vi "Shift.vi"(8 "error in":errorcluster) -> (0 "error out":errorcluster)   [LabVIEW 2015]
uses:
  Control Button/Save.ctl
  Control Button/Exit.ctl
  <vilib>/addons/database/Connection.llb/DB Tools Open Connec (String).vi
  <vilib>/addons/database/_DB Variant To Data/Database Variant To Data.xnode
  <vilib>/addons/database/NI_Database_API.lvlib
panel:
  in  "To-C 2":timestamp=timestamp(3526421399 s since 1904-01-01) format="%<%H:%M:%S\n%d/%m/%Y>T"
  in  "From-C 2":timestamp=timestamp(3526482600 s since 1904-01-01) format="%<%H:%M:%S\n%d/%m/%Y>T"
  out "error out 2":errorcluster
  out "error out":errorcluster
  out "Shift":string="B"
  in  "To-C 1":timestamp=timestamp(3526421399 s since 1904-01-01) format="%<%H:%M:%S\n%d/%m/%Y>T"
  in  "From-C 1":timestamp=timestamp(3526482600 s since 1904-01-01) format="%<%H:%M:%S\n%d/%m/%Y>T"
  in  "To-B":timestamp=timestamp(3526482599 s since 1904-01-01) format="%<%H:%M:%S\n%d/%m/%Y>T"
  in  "From-B":timestamp=timestamp(3526452000 s since 1904-01-01) format="%<%H:%M:%S\n%d/%m/%Y>T"
  in  "To-A":timestamp=timestamp(3526451999 s since 1904-01-01) format="%<%H:%M:%S\n%d/%m/%Y>T"
  in  "From-A":timestamp=timestamp(3526594200 s since 1904-01-01) format="%<%H:%M:%S\n%d/%m/%Y>T"
  in  "Exit":T1
  in  "Save":T2
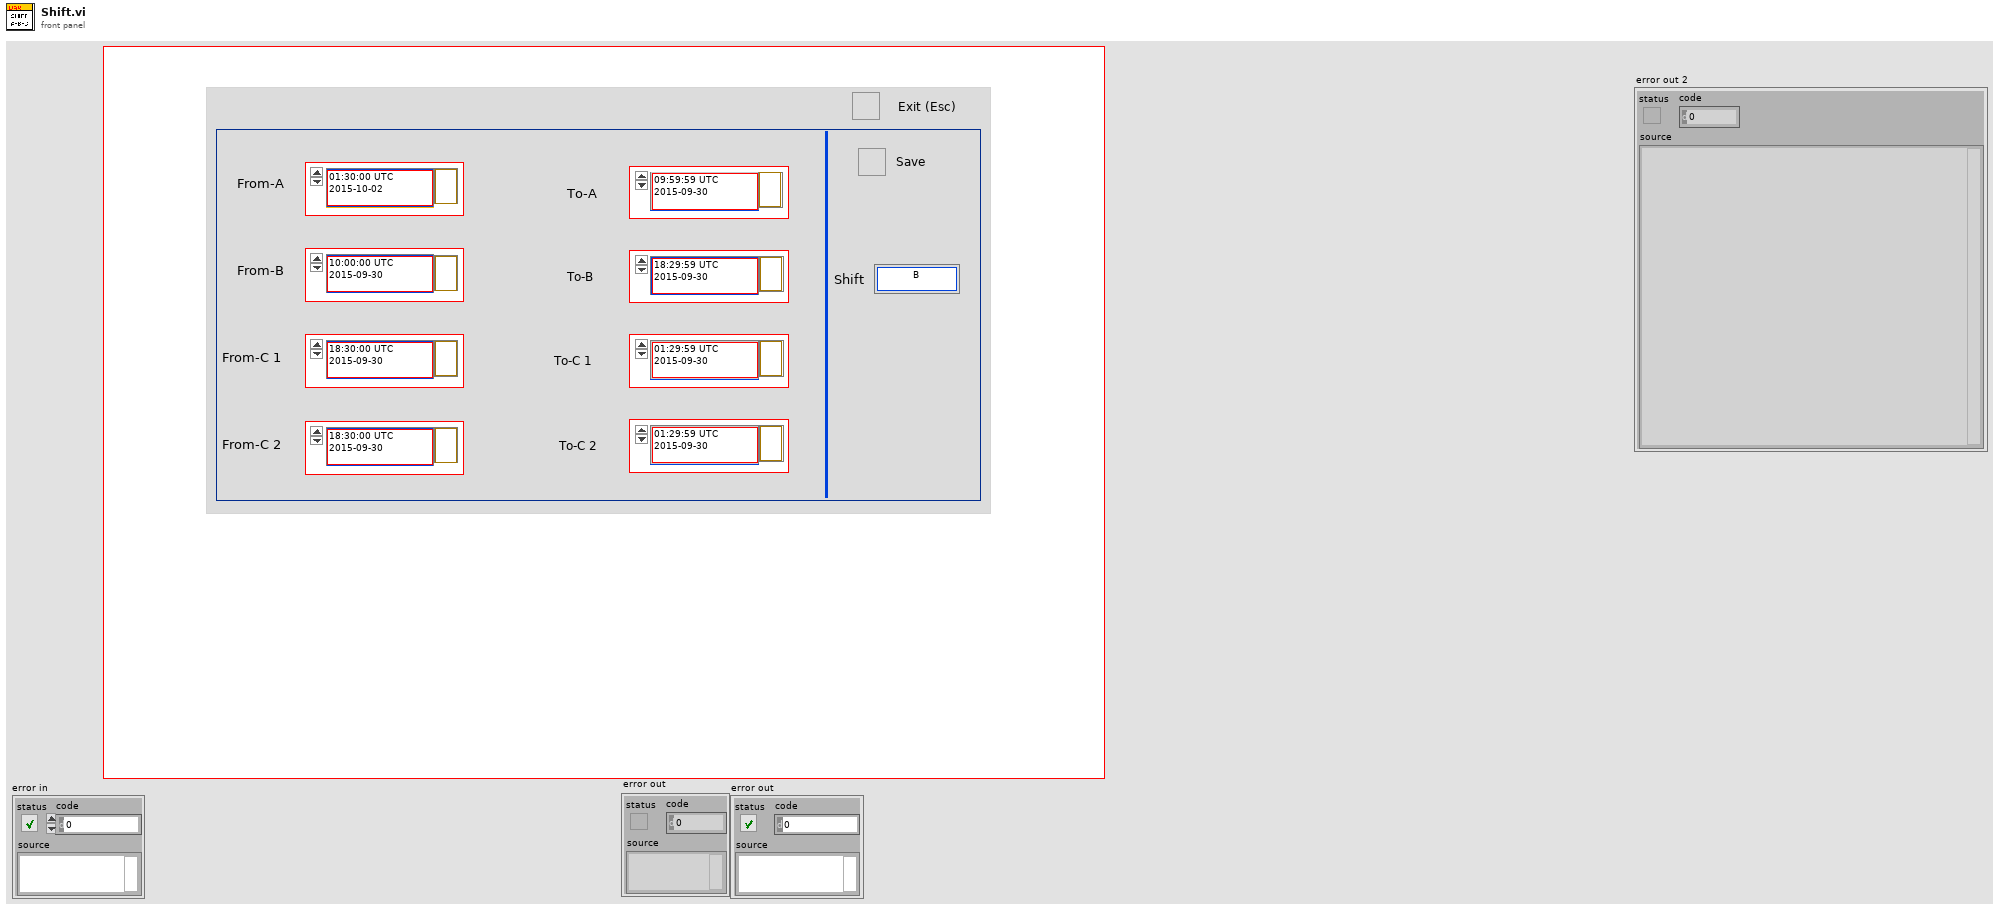
[diagram p1: front panel]
types:
  T1 = typedef "Exit.ctl" = bool
  T2 = typedef "Save.ctl" = bool
  T3 = cluster{"To-A":timestamp, "From-A":timestamp, "From-B":timestamp, "To-B":timestamp, "From-C 1":timestamp, "To-C 1":timestamp, "Shift":string, "To-C 2":timestamp, "From-C 2":timestamp}[]
  T4 = cluster{"To-A":timestamp, "From-A":timestamp, "From-B":timestamp, "To-B":timestamp, "From-C 1":timestamp, "To-C 1":timestamp, "Shift":string, "To-C 2":timestamp, "From-C 2":timestamp}
  T5 = typedef "NI_Database_API.lvlib/Conn ObjectReference.ctl" = refnum<k1>
  T6 = cluster{"To-A":timestamp, "From-A":timestamp, "From-B":timestamp, "To-B":timestamp, "From-C 1":timestamp, "To-C 1":timestamp, "From-C 2":timestamp, "To-C 2":timestamp}
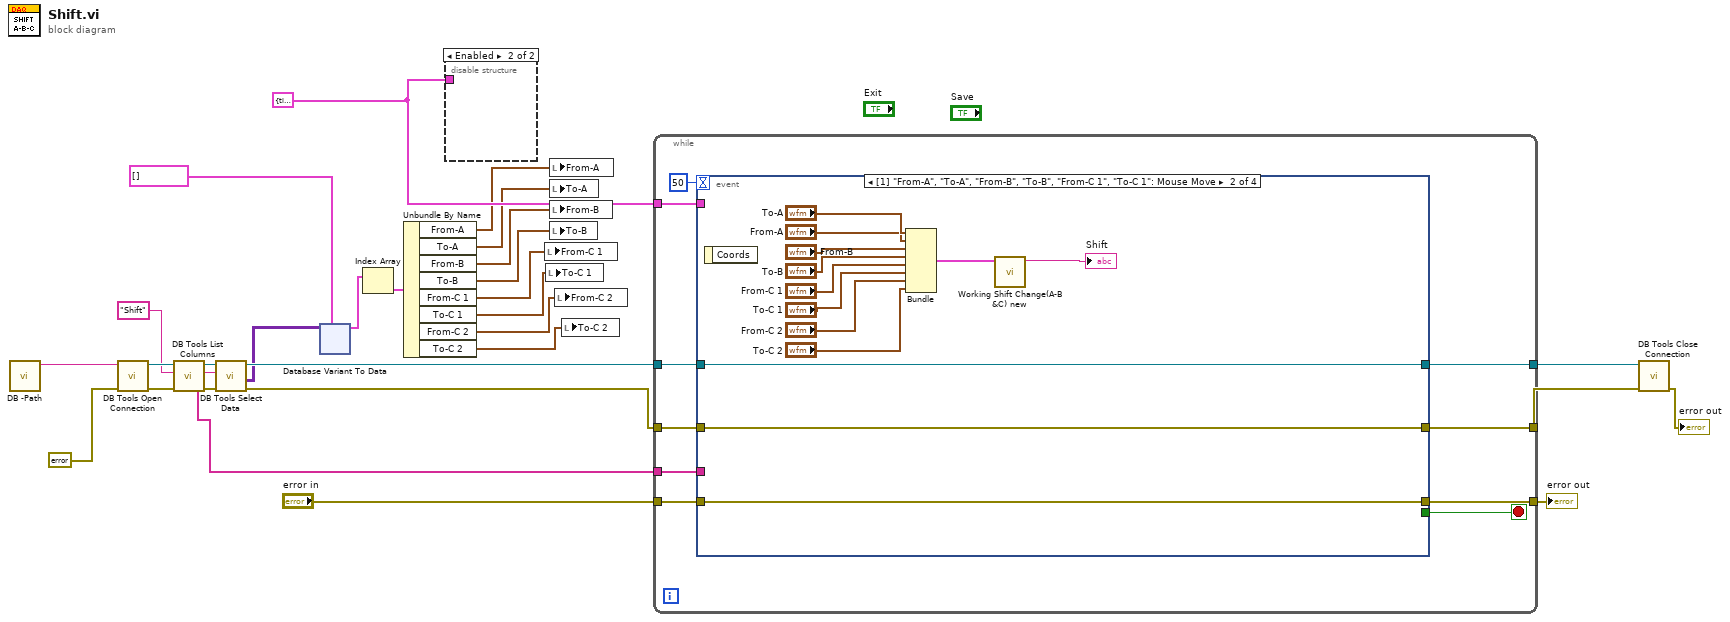
[diagram p0: block diagram]
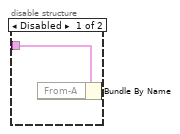
[diagram p2: hidden frame]
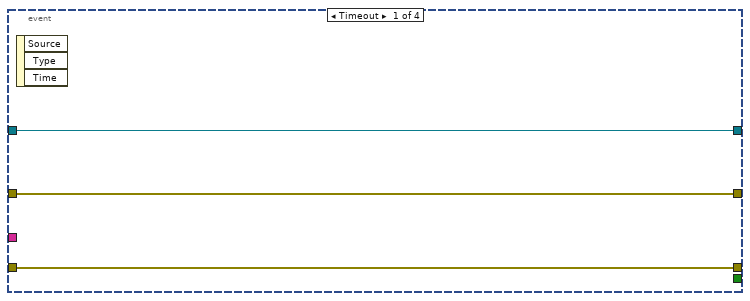
[diagram p3: hidden frame]
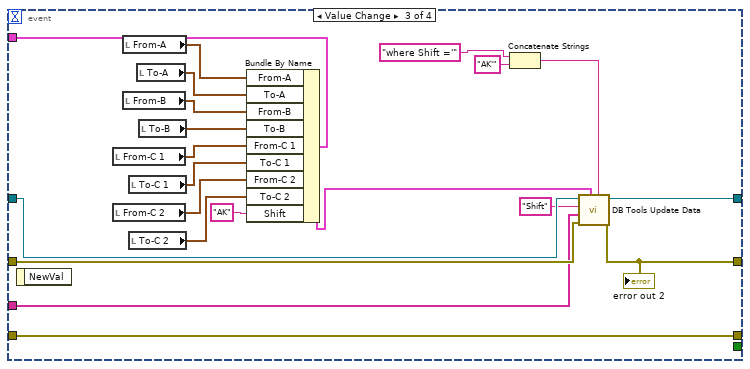
[diagram p4: hidden frame]
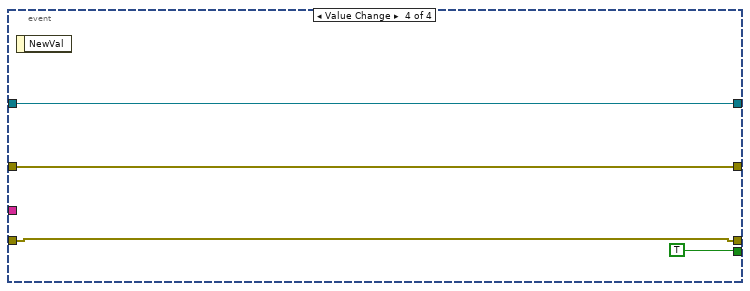
[diagram p5: hidden frame]
diagram:
  w18 = "Shift" ("table")
  w25 = T4 {"To-A"=timestamp(3526451999 s since 1904-01-01), "From-A"=timestamp(3526594200 s since 1904-01-01), "From-B"=timestamp(3526452000 s since 1904-01-01), "To-B"=timestamp(3526482599 s since 1904-01-01), "From-C 1"=timestamp(3526482600 s since 1904-01-01), "To-C 1"=timestamp(3526421399 s since 1904-01-01), "Shift"="", "To-C 2"=timestamp(3526421399 s since 1904-01-01), "From-C 2"=timestamp(3526482600 s since 1904-01-01)} ("Cluster")
  n1 = call "DB -Path.vi"() -> ("String"=w28:string)  [unwired: 11 in]
  n2 = call-poly <vilib>:"DB Tools Open Connection.vi"("error in (no error)"=errorcluster {"status"=FALSE, "code"=0, "source"=""}, "connection information"=w28) -> ("error out"=w19:errorcluster, "connection reference"=w20:T5)  [unwired: 6 in]
  n3 = call <vilib>:"DB Tools List Columns.vi"("error in (no error)"=w19, "table"=w18, "connection reference"=w20) -> ("error out"=w16:errorcluster, "columns"=w15:string[], "connection reference out"=w17:T5)  [unwired: 1 in, 1 out]
  n4 = call <vilib>:"DB Tools Select Data.vi"("error in (no error)"=w16, "table"=w18, "connection reference"=w17) -> ("error out"=w26:errorcluster, "data"=w5:variant[][], "connection reference out"=w27:T5)  [unwired: 3 in]
  n5 = xnode "Database Variant To Data"("database variant"=w5, "type"=T3 []) -> ("data"=w13:T3)  [unwired: 1 in, 1 out]
  n6 = Index Array(array=w13) -> (element=w12:T4)  [unwired: 1 in]
  n7 = Unbundle By Name(w12) -> ("From-A"=w11:timestamp, "To-A"=w10:timestamp, "From-B"=w9:timestamp, "To-B"=w8:timestamp, "From-C 1"=w7:timestamp, "To-C 1"=w6:timestamp, "From-C 2"=w2:timestamp, "To-C 2"=w1:timestamp)
  n8 = disable-structure shown="Enabled" {
    disable-tunnel: w25 -> [w29 _]
    frame Disabled {
      n9 = Bundle By Name(cluster=w29) -> ()  [unwired: 1 in, 1 out]
    }
    frame Enabled {
    }
  }
  n10 = local write "From-C 1"(w7) -> ()
  n11 = local write "To-C 1"(w6) -> ()
  n12 = local write "From-A"(w11) -> ()
  n13 = local write "To-A"(w10) -> ()
  n14 = local write "From-B"(w9) -> ()
  n15 = local write "To-B"(w8) -> ()
  n16 = local write "From-C 2"(w2) -> ()
  n17 = local write "To-C 2"(w1) -> ()
  n18 = while {
    tunnel: w27 -> [w38]
    tunnel: w26 -> [w37]
    tunnel: [w36] -> w24
    tunnel: [w35] -> w23
    tunnel: w25 -> [w34]
    tunnel: w15 -> [w33]
    tunnel: "error in" -> [w32]
    tunnel: [w31] -> w3
    stop <- w39 stop-if-true
    n19 = event shown="[1] \"From-A\", \"To-A\", \"From-B\", \"To-B\", \"From-C 1\", \"To-C 1\": Mouse Move" {
      selector: _ -> [_ _ _ _]
      dyn-events: _ -> [_ _ _ _]
      timeout: 50 -> [_ _ _ _]
      tunnel: [_ _ _ TRUE] -> w39
      tunnel: w38 -> [w41 w55 w73 w78]
      tunnel: w37 -> [w40 w54 w72 w77]
      tunnel: [w41 w55 w75 w78] -> w36
      tunnel: [w40 w54 w74 w77] -> w35
      tunnel: w34 -> [_ _ w71 _]
      tunnel: w33 -> [_ _ w59 _]
      tunnel: w32 -> [w42 w53 w58 w79]
      tunnel: [w42 w53 w58 w79] -> w31
      event Timeout {
        n20 = event-data() -> ()  [unwired: 1 in, 3 out]
      }
      event "From-A", "To-A", "From-B", "To-B", "From-C 1", "To-C 1": Mouse Move {
        n21 = event-data() -> ()  [unwired: 1 in, 1 out]
        n22 = Bundle("To-A"="To-A", "From-A"="From-A", "From-B"="From-B", "To-B"="To-B", "From-C 1"="From-C 1", "To-C 1"="To-C 1", "From-C 2"="From-C 2", "To-C 2"="To-C 2") -> (w44:T6)  [unwired: 1 in]
        n23 = call "Working Shift Change(A-B &C) new.vi"("input cluster"=w44) -> ("Shift Change"=→"Shift":string)  [unwired: 10 in]
      }
      event Value Change {
        n24 = event-data() -> ()  [unwired: 1 in, 1 out]
        n25 = local read "From-C 1"() -> (w66:timestamp)
        n26 = local read "From-C 2"() -> (w57:timestamp)
        n27 = local read "From-A"() -> (w70:timestamp)
        n28 = local read "From-B"() -> (w68:timestamp)
        n29 = local read "To-C 1"() -> (w65:timestamp)
        n30 = local read "To-C 2"() -> (w56:timestamp)
        n31 = local read "To-A"() -> (w69:timestamp)
        n32 = local read "To-B"() -> (w67:timestamp)
        n33 = Bundle By Name(cluster=w71, "From-A"=w70, "To-A"=w69, "From-B"=w68, "To-B"=w67, "From-C 1"=w66, "To-C 1"=w65, "From-C 2"=w57, "To-C 2"=w56, "Shift"="AK") -> (w76:T4)
        n34 = Concatenate Strings("where Shift ='" ("string"), "AK'" ("string")) -> (w60:string)
        n35 = call <vilib>:"DB Tools Update Data.vi"("condition"=w60, "data"=w76, "error in (no error)"=w72, "columns"=w59, "table"="Shift", "connection reference"=w73) -> ("error out"=w74:errorcluster, "connection reference out"=w75:T5)  [unwired: 4 in]
        "error out 2" <- w74
      }
      event Value Change {
        n36 = event-data() -> ()  [unwired: 1 in, 1 out]
      }
    }
  }
  "error out" <- w3
  n37 = call <vilib>:"DB Tools Close Connection.vi"("error in (no error)"=w23, "connection reference"=w24) -> ("error out"=→"error out":errorcluster)  [unwired: 5 in]
